vi "Read refnum.vi"(8 "error in (no error)":errorcluster, 11 "INIFileClass in":refnum<class "INIFileClass.lvclass">) -> (0 "error out":errorcluster, 2 "config data":T1, 3 "INIFileClass out":refnum<class "INIFileClass.lvclass">)   [LabVIEW 2013, in "INIFileClass.lvclass"]
uses:
  INIFileClass.lvclass
  <vilib>/Utility/config.llb/Config Data RefNum.ctl
  INIFileClass.lvclass/INIFileClass.ctl
  <vilib>/Utility/config.llb/NI_LVConfig.lvlib
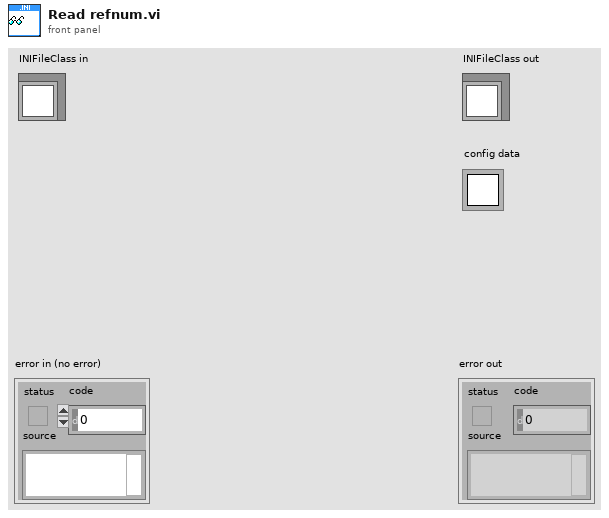
[diagram p1: front panel]
types:
  T1 = typedef "NI_LVConfig.lvlib/Config Data RefNum.ctl" = refnum<k1>
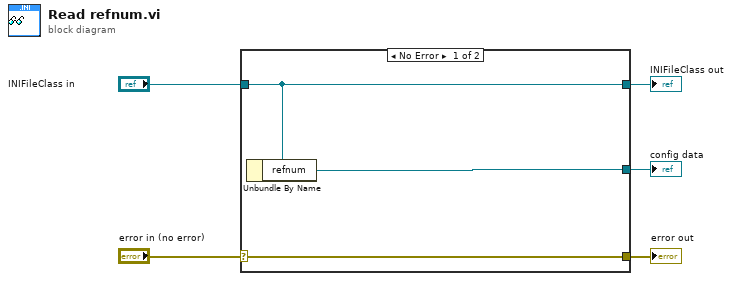
[diagram p0: block diagram]
diagram:
  n1 = case shown="No Error" "error in (no error)" {
    selector: "error in (no error)" -> [w8 w9]
    tunnel: [w8 w9] -> w4
    tunnel: [w7 w10] -> w2
    tunnel: "INIFileClass in" -> [w7 w10]
    tunnel: [w6 _] -> w1
    frame No Error {
      n2 = Unbundle By Name(w7) -> ("refnum"=w6:T1)
    }
    frame Error {
    }
  }
  "error out" <- w4
  "INIFileClass out" <- w2
  "config data" <- w1
